vi "analysis_images2.vi"() -> ()   [LabVIEW 2019]
uses:
  <vilib>/gmath/NI_Gmath.lvlib
  <vilib>/Analysis/NI_AALBase.lvlib
panel:
  out "size(s)":i32
  out "CV":dbl
  out "variance":dbl format="%0.2f"
  out "standard deviation":dbl format="%0.2f"
  out "mean":dbl format="%0.2f"
  out "XY Graph 6":cluster{timestamp[], dbl[]}(graph)
  out "element":timestamp
  in  "Repeats":bool
  in  "Controls":bool
  out "XY Graph 4":cluster{dbl, "Numeric":dbl}[](graph)
  out "XY Graph 3":cluster{"Best Linear Fit":dbl[], dbl[]}[](graph)
  out "XY Graph 2":cluster{dbl, "Numeric":dbl}[](graph)
  out "XY Graph":cluster{dbl[], "Y":dbl[]}[](graph)
  in  "directory path":path
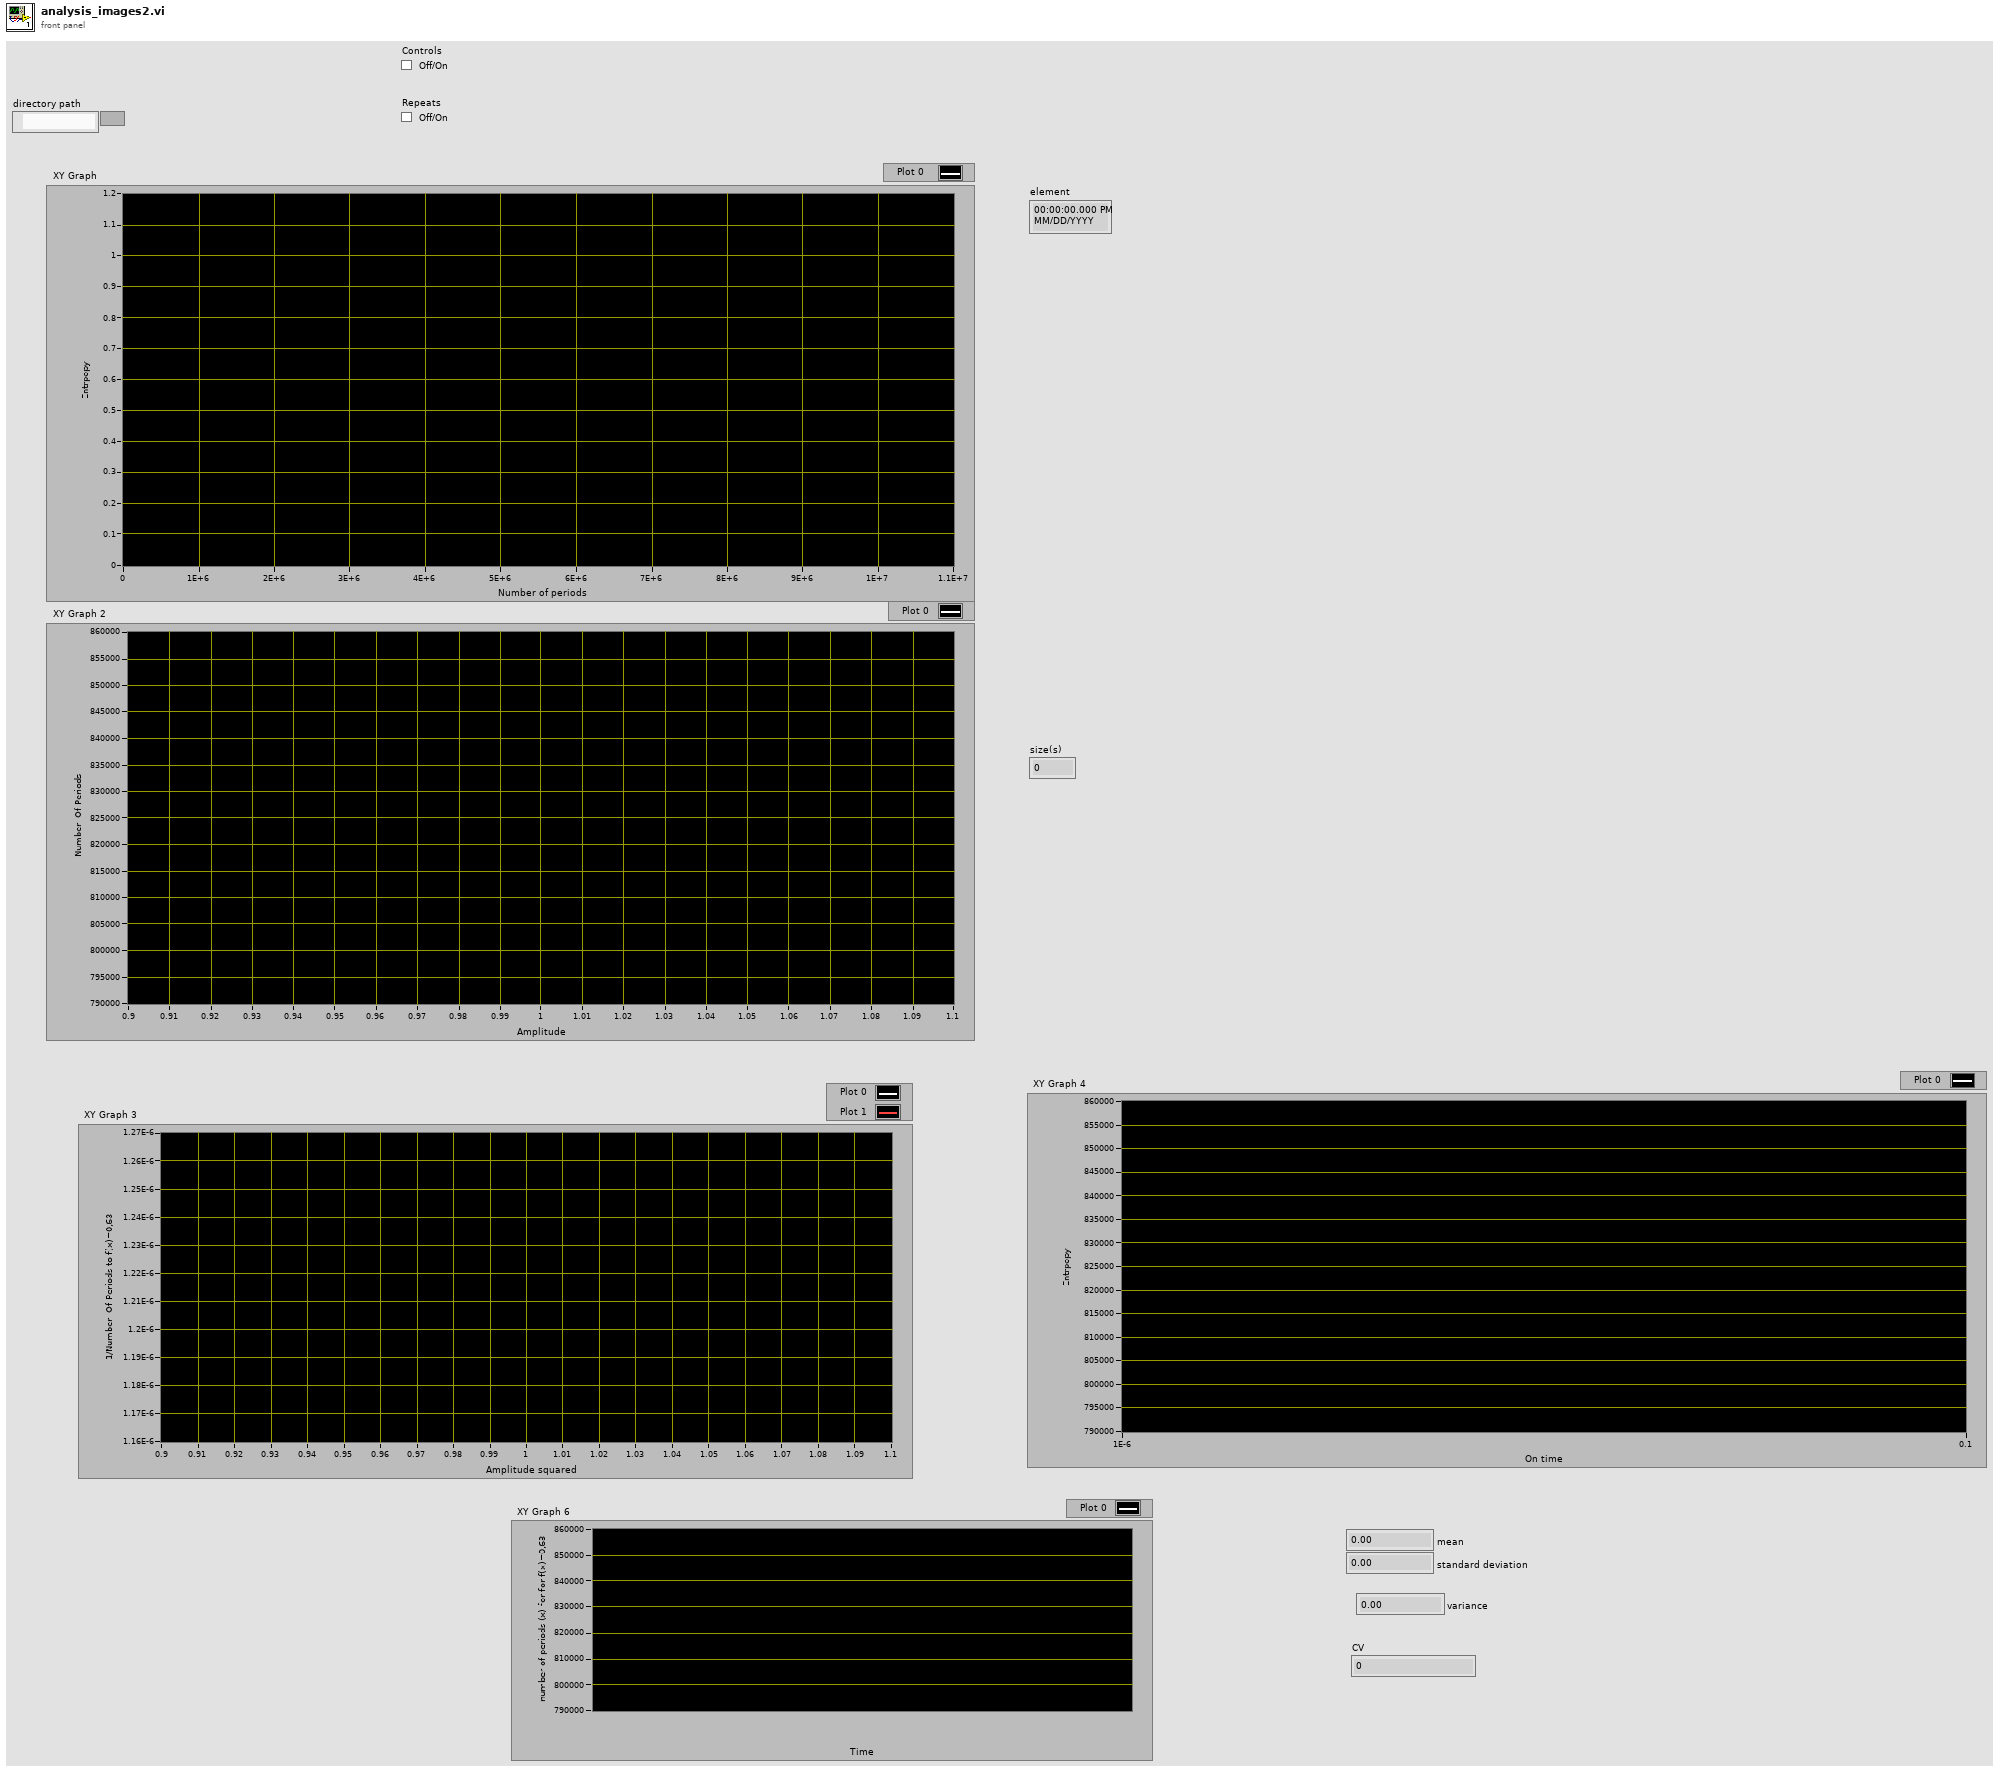
[diagram p1: front panel]
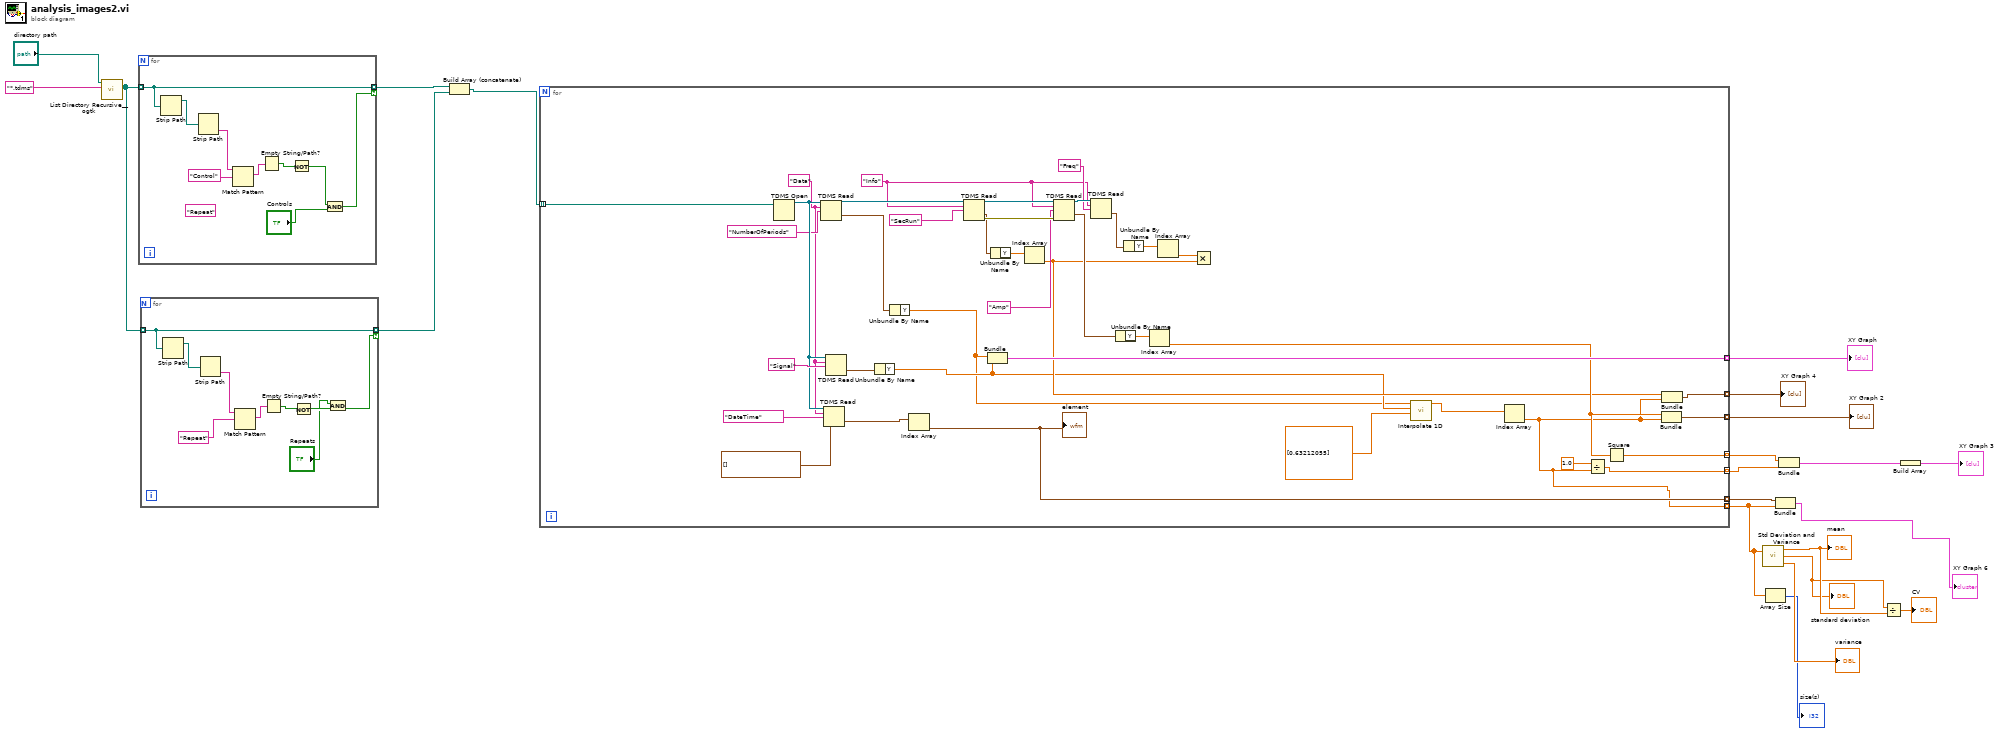
[diagram p0: block diagram]
diagram:
  n1 = call <userlib>:"List Directory Recursive__ogtk.vi"("pattern"="*.tdms", "Path"="directory path") -> ("file paths"=w12:path[])  [unwired: 6 in, 3 out]
  n2 = for {
    tunnel: w12 -> [w27] mode=indexing
    tunnel: [w27] -> w10 mode=indexing if=w22
    (unwired) "Repeat" ("group name in")
    n3 = Strip Path(path=w27) -> (stripped path=w30:path)  [unwired: 1 out]
    n4 = Strip Path(path=w30) -> (name=w29:string)  [unwired: 1 out]
    n5 = Match Pattern(string=w29, regular expression="Control" ("group name in")) -> (match substring=w28:string)  [unwired: 1 in, 3 out]
    n6 = Empty String/Path?(string/path=w28) -> (empty?=w26:bool)
    n7 = Not(x=w26) -> (.not. x?=w23:bool)
    n8 = And(x=w23, y="Controls") -> (x .and. y?=w22:bool)
  }
  n9 = for {
    tunnel: w12 -> [w36] mode=indexing
    tunnel: [w36] -> w9 mode=indexing if=w32
    n10 = Strip Path(path=w36) -> (stripped path=w39:path)  [unwired: 1 out]
    n11 = Strip Path(path=w39) -> (name=w38:string)  [unwired: 1 out]
    n12 = Match Pattern(string=w38, regular expression="Repeat" ("group name in")) -> (match substring=w37:string)  [unwired: 1 in, 3 out]
    n13 = Empty String/Path?(string/path=w37) -> (empty?=w35:bool)
    n14 = Not(x=w35) -> (.not. x?=w34:bool)
    n15 = And(x="Repeats", y=w34) -> (x .and. y?=w32:bool)
  }
  n16 = Build Array (concatenate)(w10, w9) -> (w11:path[])
  n17 = for {
    tunnel: [w73] -> w19 mode=indexing
    tunnel: [w66] -> w18 mode=indexing
    tunnel: w11 -> [w65] mode=indexing
    tunnel: [w61] -> w17 mode=indexing
    tunnel: [w42] -> w16 mode=indexing
    tunnel: [w52] -> w13 mode=indexing
    tunnel: [w44] -> w8 mode=indexing
    tunnel: [w43] -> w2 mode=indexing
    w51 = "Info" ("group name in")
    w48 = "Data" ("group name in")
    n18 = TDMS Open(11:w65) -> (3:w50:refnum<k34>)  [unwired: 6 in, 1 out]
    n19 = TDMS Read(0:w50, 5:w48, 7:"NumberOfPeriods" ("group name in")) -> (4:w77:refnum<k34>, 10:w78:waveform(dbl))  [unwired: 5 in, 4 out]
    n20 = TDMS Read(0:w50, 5:w48, 7:"DateTime" ("group name in"), 12:timestamp[] []) -> (10:w46:timestamp[])  [unwired: 4 in, 5 out]
    n21 = TDMS Read(0:w50, 5:w48, 7:"Signal" ("group name in")) -> (10:w75:waveform(dbl))  [unwired: 5 in, 5 out]
    n22 = Unbundle By Name(w75) -> ("Y"=w41:dbl[])
    n23 = Unbundle By Name(w78) -> ("Y"=w40:dbl[])
    n24 = Index Array(array=w46) -> (element=w44:timestamp)  [unwired: 1 in]
    "element" <- w44
    n25 = TDMS Read(0:w77, 5:w51, 7:"SecRun" ("group name in")) -> (4:w71:refnum<k34>, 10:w55:waveform(dbl), 15:w70:errorcluster)  [unwired: 5 in, 3 out]
    n26 = Bundle("Y"=w40, "Y"=w41) -> (w73:cluster{"Y":dbl[], "Y":dbl[]})  [unwired: 1 in]
    n27 = Unbundle By Name(w55) -> ("Y"=w56:dbl[])
    n28 = Index Array(array=w56) -> (element=w53:dbl)  [unwired: 1 in]
    n29 = TDMS Read(0:w71, 5:w51, 7:"Amp" ("group name in"), 11:w70) -> (4:w60:refnum<k34>, 10:w68:waveform(dbl))  [unwired: 4 in, 4 out]
    n30 = TDMS Read(0:w60, 5:w51, 7:"Freq" ("group name in")) -> (10:w57:waveform(dbl))  [unwired: 5 in, 5 out]
    n31 = Unbundle By Name(w68) -> ("Y"=w67:dbl[])
    n32 = Unbundle By Name(w57) -> ("Y"=w58:dbl[])
    n33 = Index Array(array=w67) -> (element=w63:dbl)  [unwired: 1 in]
    n34 = Index Array(array=w58) -> (element=w54:dbl)  [unwired: 1 in]
    n35 = Multiply(x=w54, y=w53) -> ()  [unwired: 1 out]
    n36 = call <vilib>:"Interpolate 1D.vi"("xi"=dbl[] [0.63212055], "X"=w41, "Y"=w40) -> ("yi"=w64:dbl[])  [unwired: 6 in, 2 out]
    n37 = Index Array(array=w64) -> (element=w43:dbl)  [unwired: 1 in]
    n38 = Divide(x=1.0, y=w43) -> (x/y=w42:dbl)
    n39 = Square(x=w63) -> (x^2=w61:dbl)
    n40 = Bundle(w63, "Numeric"=w43) -> (w66:cluster{dbl, "Numeric":dbl})  [unwired: 1 in]
    n41 = Bundle(w53, "Numeric"=w43) -> (w52:cluster{dbl, "Numeric":dbl})  [unwired: 1 in]
  }
  "XY Graph" <- w19
  "XY Graph 2" <- w18
  "XY Graph 4" <- w13
  n42 = call <vilib>:"Std Deviation and Variance.vi"("X"=w2) -> ("mean"=w4:dbl, "standard deviation"=w3:dbl, "variance"=→"variance":dbl)  [unwired: 1 in]
  "mean" <- w4
  "standard deviation" <- w3
  n43 = Array Size(array=w2) -> (size(s)=→"size(s)":i32)
  n44 = Bundle(w8, w2) -> (→"XY Graph 6":cluster{timestamp[], dbl[]})  [unwired: 1 in]
  n45 = Bundle(w17, w16) -> (w15:cluster{dbl[], dbl[]})  [unwired: 1 in]
  n46 = Divide(x=w3, y=w4) -> (x/y=→"CV":dbl)
  n47 = Build Array(w15) -> (→"XY Graph 3":cluster{dbl[], dbl[]}[])
